vi "Position Done Key.vi"(8 "error in (no error)":errorcluster, 10 "Space Bar Key":refnum<vi>, 11 "Done Key":refnum<vi>) -> (0 "error out":errorcluster)   [LabVIEW 2014]
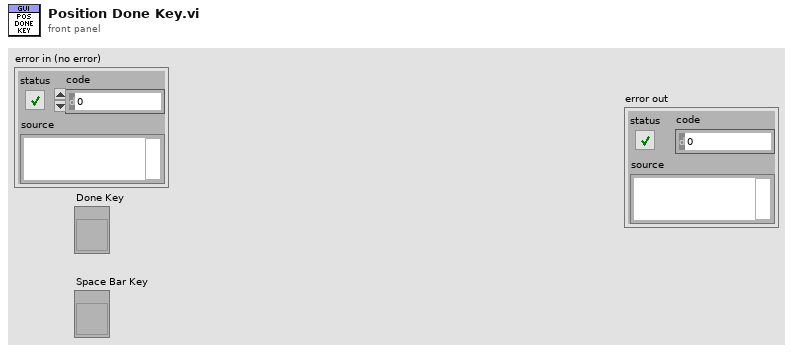
[diagram p1: front panel]
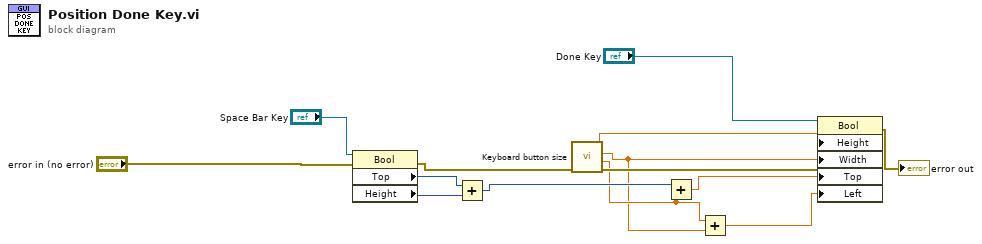
[diagram p0: block diagram]
diagram:
  n1 = property class="Bool"(reference="Space Bar Key", error in="error in (no error)") -> (error out=w10:errorcluster, "Top"=w8:i32, "Height"=w7:u32)  [unwired: 1 out]
  n2 = Add(x=w8, y=w7) -> (x+y=w6:u32)
  n3 = call "Keyboard button size.vi"("error in (no error)"=w10) -> ("error out"=w13:errorcluster, "Key Spacing"=w3:dbl, "Key Width"=w2:dbl, "Key Height"=w11:dbl)  [unwired: 7 in]
  n4 = Add(x=w6, y=w3) -> (x+y=w5:dbl)
  n5 = Add(x=w3, y=w2) -> (x+y=w1:dbl)
  n6 = property class="Bool"(reference="Done Key", error in=w13, "Height"=w11, "Width"=w2, "Top"=w5, "Left"=w1) -> (error out=→"error out":errorcluster)  [unwired: 1 out]
